vi "measurementSetupPanel.vi"() -> ()   [LabVIEW 2017]
uses:
  Controls/chanType.ctl
  Globals/measurementGlobal.vi
panel:
  in  "Submission Button":bool
  in  "Pressure Scanner Clock Chans.":T1(array[cluster])
  in  "Channel Info.":T3(array[cluster])
  in  "Input No of Blocks":i32
  in  "Input No of samples":i32
  in  "Input Sampling rate (Hz)":dbl
  in  "NI Device Name":enum16{"USB-6210", "USB-6218"}(ring)
  in  "Acquisition Cards":enum16{"NI-USB-6210_Kernel.vi"}(ring)
  in  "Setup":enum16{"Run Programme", "Show Setup"}(ring)
  # "- Add calibration file path\n- Add lab atmospheric information such as (P, T)"
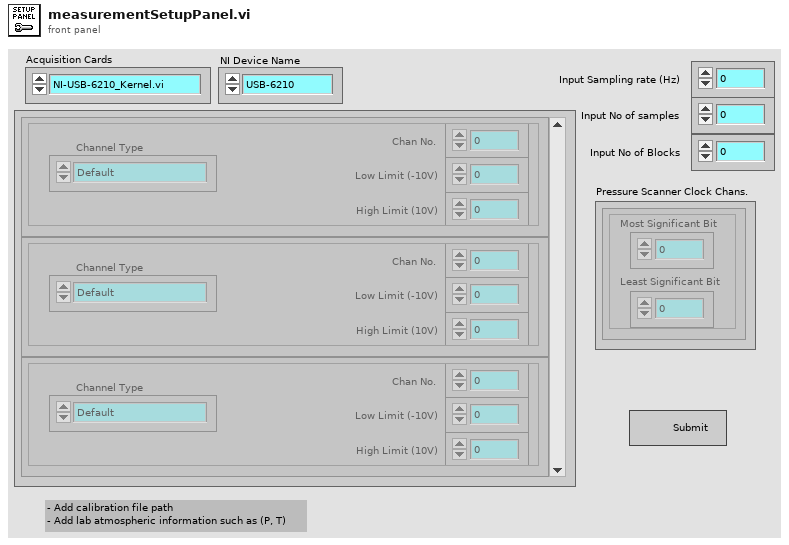
[diagram p1: front panel]
types:
  T1 = cluster{"Least Significant Bit":dbl, "Most Significant Bit":dbl}[]
  T2 = typedef "chanType.ctl" = enum16{"Default", "Clock", "Pressure Scanner"}
  T3 = cluster{"Channel Type":T2, "Chan No.":i32, "Low Limit (-10V)":dbl, "High Limit (10V)":dbl}[]
  T4 = enum32{"Invalid", "Standard", "Closed", "Hidden", "Minimized", "Maximized"}
  T5 = typedef "chan&Span.ctl" = cluster{"Chan No.":i32, "Low Volt Limit (-10V)":dbl, "High Volt Limit (10V)":dbl, "input terminal configuration":i32}
  T6 = cluster{"Most Significant Bit":dbl, "Least Significant Bit":dbl}[]
  T7 = cluster{"Most Significant Bit":dbl, "Least Significant Bit":dbl}
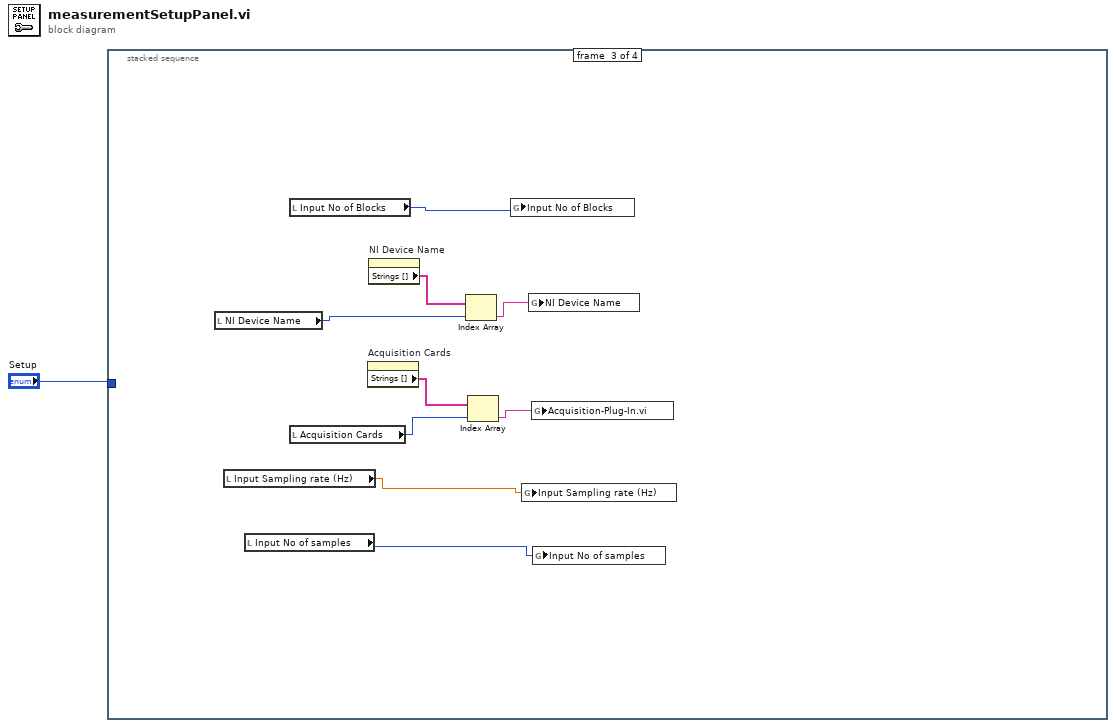
[diagram p0: block diagram]
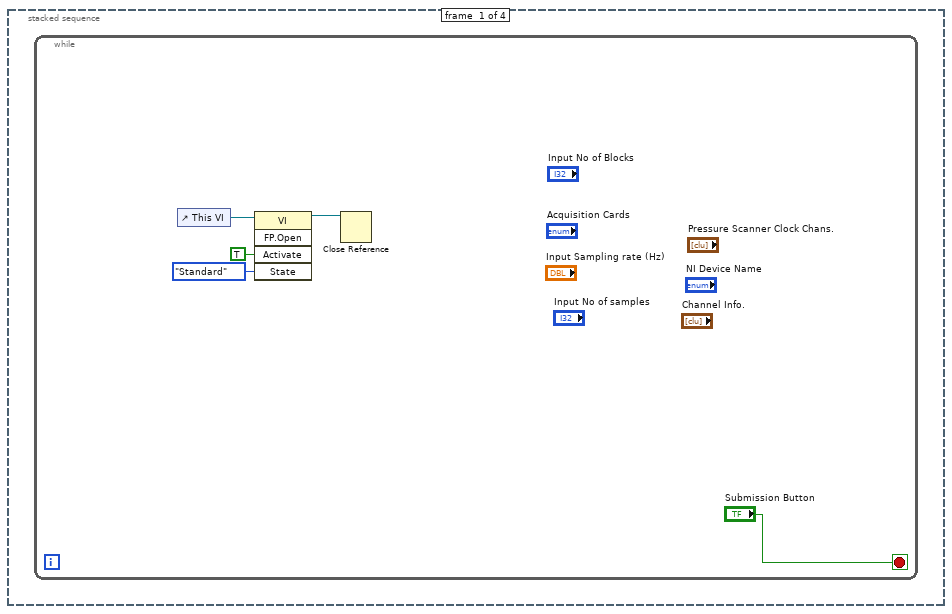
[diagram p2: hidden frame]
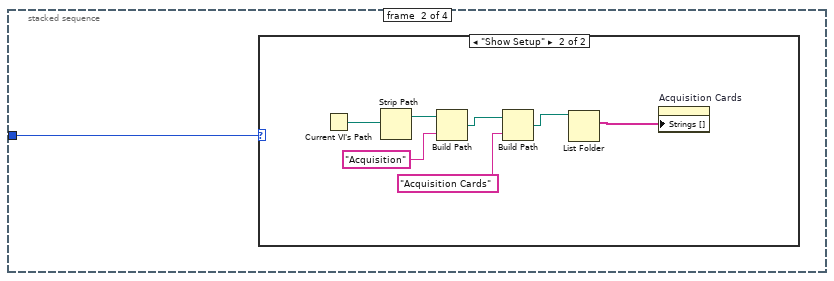
[diagram p3: hidden frame]
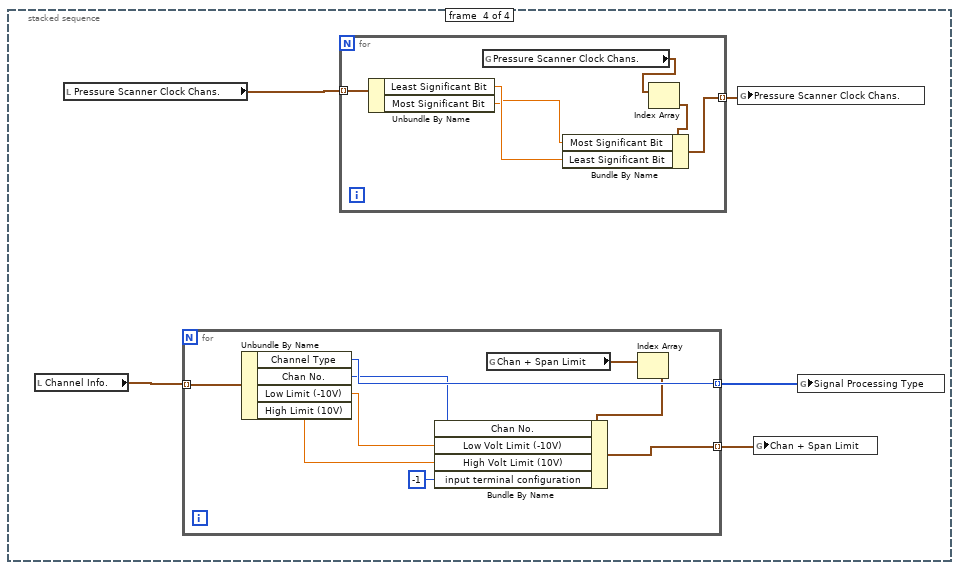
[diagram p5: hidden frame]
diagram:
  n1 = stacked-sequence {
    tunnel: "Setup" -> [_ w7 _ _]
    frame #0 {
      n2 = while {
        stop <- "Submission Button" stop-if-true
        n3 = control-ref of="This VI"() -> (w4:refnum<vi>)
        n4 = invoke class="VI" method="FP.Open"(reference=w4, "Activate"=TRUE ("Activate?"), "State"=T4."Standard") -> (reference out=w3:refnum<vi>)  [unwired: 2 in, 4 out]
        n5 = Close Reference(reference=w3) -> ()  [unwired: 1 in, 1 out]
      }
    }
    frame #1 {
      n6 = case shown="\"Show Setup\"" w7 {
        frame "Run Programme", Default {
        }
        frame "Show Setup" {
          n7 = Current VI's Path() -> (path=w14:path)
          n8 = Strip Path(path=w14) -> (stripped path=w13:path)  [unwired: 1 out]
          n9 = Build Path(base path=w13, name or relative path="Acquisition") -> (appended path=w11:path)
          n10 = Build Path(base path=w11, name or relative path="Acquisition Cards") -> (appended path=w9:path)
          n11 = List Folder(path=w9) -> (filenames=w8:string[])  [unwired: 3 in, 3 out]
          n12 = property on="Acquisition Cards" class="Enum (strict)"("Strings []"=w8) -> ()  [unwired: 2 in, 2 out]
        }
      }
    }
    frame #2 {
      n13 = local read "NI Device Name"() -> (w17:enum16{"USB-6210", "USB-6218"})
      n14 = local read "Input Sampling rate (Hz)"() -> (w16:dbl)
      n15 = local read "Input No of samples"() -> (w15:i32)
      n16 = local read "Input No of Blocks"() -> (w18:i32)
      n17 = local read "Acquisition Cards"() -> (w19:enum16{"NI-USB-6210_Kernel.vi"})
      n18 = property on="Acquisition Cards" class="Enum (strict)"() -> ("Strings []"=w23:string[])  [unwired: 2 in, 2 out]
      n19 = property on="NI Device Name" class="Enum (strict)"() -> ("Strings []"=w21:string[])  [unwired: 2 in, 2 out]
      n20 = Index Array(array=w21, index=w17) -> (element=w20:string)
      n21 = Index Array(array=w23, index=w19) -> (element=w22:string)
      n22 = global write "measurementGlobal.vi" "Input No of Blocks"(w18) -> ()
      n23 = global write "measurementGlobal.vi" "Input Sampling rate (Hz)"(w16) -> ()
      n24 = global write "measurementGlobal.vi" "NI Device Name"(w20) -> ()
      n25 = global write "measurementGlobal.vi" "Acquisition-Plug-In.vi"(w22) -> ()
      n26 = global write "measurementGlobal.vi" "Input No of samples"(w15) -> ()
    }
    frame #3 {
      n27 = local read "Channel Info."() -> (w24:T3)
      n28 = local read "Pressure Scanner Clock Chans."() -> (w25:T1)
      n29 = for {
        tunnel: w24 -> [w43] mode=indexing
        tunnel: [w42] -> w28 mode=indexing
        tunnel: [w36] -> w26 mode=indexing
        n30 = Unbundle By Name(w43) -> ("Channel Type"=w42:T2, "Chan No."=w41:i32, "Low Limit (-10V)"=w40:dbl, "High Limit (10V)"=w39:dbl)
        n31 = global read "measurementGlobal.vi" "Chan + Span Limit"() -> (w38:T5[])
        n32 = Index Array(array=w38) -> (element=w37:T5)  [unwired: 1 in]
        n33 = Bundle By Name(cluster=w37, "Chan No."=w41, "Low Volt Limit (-10V)"=w40, "High Volt Limit (10V)"=w39, "input terminal configuration"=-1) -> (w36:T5)
      }
      n34 = for {
        tunnel: w25 -> [w34] mode=indexing
        tunnel: [w31] -> w27 mode=indexing
        n35 = Unbundle By Name(w34) -> ("Least Significant Bit"=w33:dbl, "Most Significant Bit"=w32:dbl)
        n36 = global read "measurementGlobal.vi" "Pressure Scanner Clock Chans."() -> (w30:T6)
        n37 = Index Array(array=w30) -> (element=w29:T7)  [unwired: 1 in]
        n38 = Bundle By Name(cluster=w29, "Most Significant Bit"=w32, "Least Significant Bit"=w33) -> (w31:T7)
      }
      n39 = global write "measurementGlobal.vi" "Pressure Scanner Clock Chans."(w27) -> ()
      n40 = global write "measurementGlobal.vi" "Chan + Span Limit"(w26) -> ()
      n41 = global write "measurementGlobal.vi" "Signal Processing Type"(w28) -> ()
    }
  }
